vi "Read GPIO Timestamps From Disk.vi"(0 "file path":path, 11 "error in (no error)":errorcluster) -> (4 "gpio timestamps":T1[](array[typedef]), 15 "error out":errorcluster)   [LabVIEW 2023, in "GettingStarted_Common_148X_Host.lvlib"]
uses:
  GettingStarted_Common_148X_Host.lvlib
  <instrlib>/FlexRIO/CSI-2/v2/Host/Types/Host GPIO Bank Timestamp.ctl
  <instrlib>/FlexRIO/CSI-2/v2/FPGA/Types/Timestamp ID.ctl
  <instrlib>/FlexRIO/CSI-2/v2/FPGA/Types/GPIO Bank.ctl
  <instrlib>/FlexRIO/CSI-2/v2/FPGA/Types/Raw Timestamp.ctl
  <instrlib>/FlexRIO/CSI-2/v2/Host/subVIs/Convert Raw Timestamp to GPIO Bank Timestamp.vi
  <instrlib>/FlexRIO/CSI-2/v2/FPGA/NI CSI-2 API FPGA v2.lvlib
  <instrlib>/FlexRIO/CSI-2/v2/Host/NI CSI-2 API Host v2.lvlib
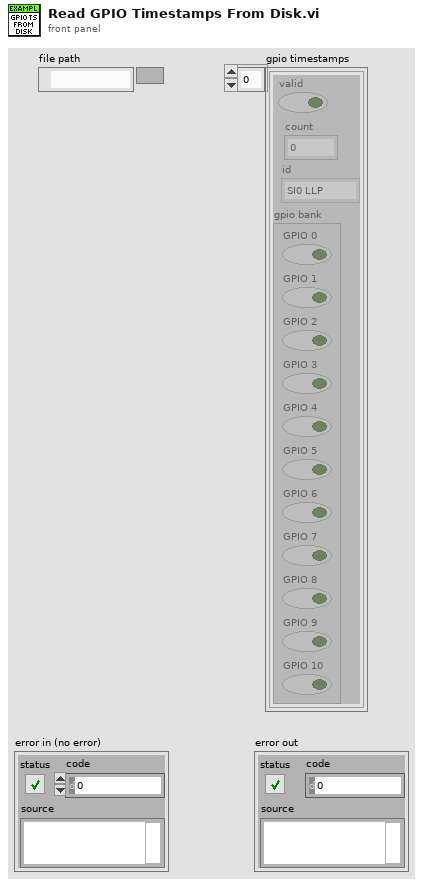
[diagram p1: front panel]
types:
  T1 = typedef "NI CSI-2 API Host v2.lvlib/Host GPIO Bank Timestamp.ctl" = cluster{"valid":bool, "count":u64, "id":T2, "gpio bank":T3}
  T2 = typedef "NI CSI-2 API FPGA v2.lvlib/Timestamp ID.ctl" = enum8{"SI0 LLP", "SI1 LLP", "SI2 LLP", "SI3 LLP", "SI4 LLP", "SI5 LLP", "SI6 LLP", "SI7 LLP", "SO0 LLP", "SO1 LLP", "SO2 LLP", "SO3 LLP", "SO4 LLP", "SO5 LLP", "SO6 LLP", "SO7 LLP", "Ser0 GPIO Bank", "Ser1 GPIO Bank", "Ser2 GPIO Bank", "Ser3 GPIO Bank", "Ser4 GPIO Bank", "Ser5 GPIO Bank", "Ser6 GPIO Bank", "Ser7 GPIO Bank", "Des0 GPIO Bank", "Des1 GPIO Bank", "Des2 GPIO Bank", "Des3 GPIO Bank", "Des4 GPIO Bank", "Des5 GPIO Bank", "Des6 GPIO Bank", "Des7 GPIO Bank", "User0", "User1", "User2", "User3", "User4", "User5", "User6", "User7", "User8", "User9", "User10", "User11", "User12", "User13", "User14", "User15", "User16", "User17", "User18", "User19", "User20", "User21", "User22", "User23", "User24", "User25", "User26", "User27", "User28", "User29", "User30", "User31"}
  T3 = typedef "NI CSI-2 API FPGA v2.lvlib/GPIO Bank.ctl" = cluster{"GPIO 0":bool, "GPIO 1":bool, "GPIO 2":bool, "GPIO 3":bool, "GPIO 4":bool, "GPIO 5":bool, "GPIO 6":bool, "GPIO 7":bool, "GPIO 8":bool, "GPIO 9":bool, "GPIO 10":bool}
  T4 = enum16{"open", "open or create", "create or replace", "create", "open (read-only)"}
  T5 = typedef "NI CSI-2 API FPGA v2.lvlib/Raw Timestamp.ctl" = cluster{"timestamp":u64, "valid":bool}
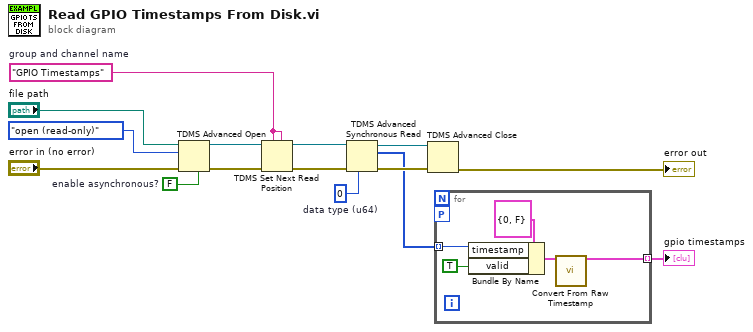
[diagram p0: block diagram]
diagram:
  w1 = "GPIO Timestamps"  # group and channel name
  w7 = FALSE  # enable asynchronous?
  w13 = u64 0  # data type (u64)
  n1 = TDMS Advanced Open(4:w7, 8:"error in (no error)", 10:T4."open (read-only)" ("operation (0:open)"), 11:"file path") -> (0:w5:errorcluster, 3:w2:refnum<k34>)  [unwired: 1 in, 1 out]
  n2 = TDMS Set Next Read Position(5:w1, 7:w1, 8:w5, 11:w2) -> (0:w4:errorcluster, 3:w3:refnum<k34>)  [unwired: 2 in]
  n3 = TDMS Advanced Synchronous Read(6:w13, 8:w4, 11:w3) -> (0:w14:errorcluster, 2:w8:u64[], 3:w15:refnum<k34>)  [unwired: 1 in, 1 out]
  n4 = TDMS Advanced Close(8:w14, 11:w15) -> (0:→"error out":errorcluster)  [unwired: 2 in, 1 out]
  n5 = for {
    tunnel: w8 -> [w18] mode=indexing
    tunnel: [w17] -> w6 mode=indexing
    workers-P: _ -> [_]
    n6 = Bundle By Name(cluster=T5 {"timestamp"=0, "valid"=FALSE} ("raw timestamp"), "timestamp"=w18, "valid"=TRUE) -> (w19:T5)
    n7 = call-poly <instrlib>:"Convert From Raw Timestamp.vi"("raw timestamp"=w19) -> ("gpio bank timestamp"=w17:T1)  [unwired: 14 in]
  }
  "gpio timestamps" <- w6
